vi "SymmetricalComponents_src.vi"(0 "A":T1, 5 "B":T1, 7 "C":T1) -> (4 "zero":T1, 6 "positive":T1, 8 "negative":T1)   [LabVIEW 2015]
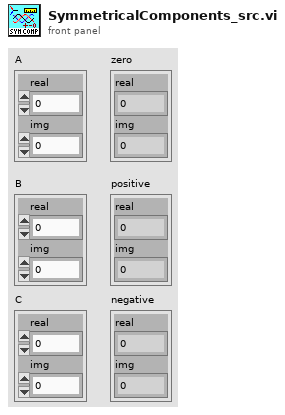
[diagram p1: front panel]
types:
  T1 = typedef "ComplexSGL" = cluster{"real":sgl, "img":sgl}
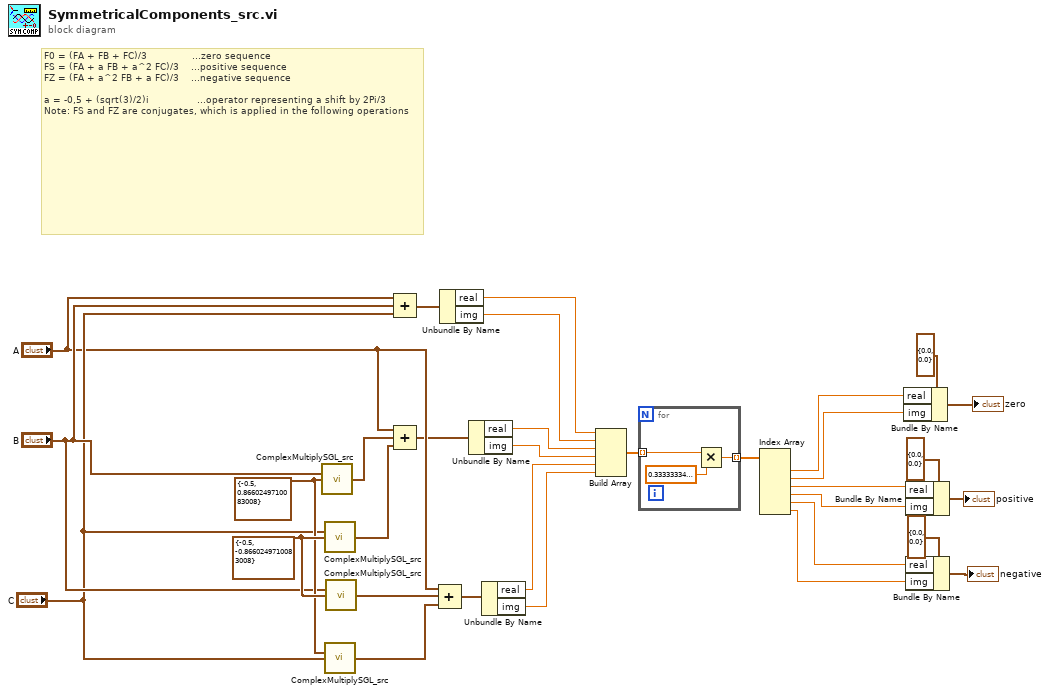
[diagram p0: block diagram]
diagram:
  w26 = T1 {"real"=-0.5, "img"=-0.866025} ("Y")
  w25 = T1 {"real"=-0.5, "img"=0.866025} ("Y")
  # "F0 = (FA + FB + FC)/3               ...zero sequence\nFS = (FA + a FB + a^2 FC)/3    ...positive sequence\nFZ = (FA + a^2 FB + a FC)/3    ...negative sequence\n\na = -0,5 + (sqrt(3)/2)i                ...operator representing a shift by 2Pi/3\nNote: FS and FZ are conjugates, which is applied in the following operations"
  n1 = call "ComplexMultiplySGL_src.vi"("X"="B", "Y"=w25) -> ("Z"=w11:T1)  [unwired: 13 in]
  n2 = call "ComplexMultiplySGL_src.vi"("X"="C", "Y"=w26) -> ("Z"=w10:T1)  [unwired: 13 in]
  n3 = call "ComplexMultiplySGL_src.vi"("X"=w25, "Y"="C") -> ("Z"=w7:T1)  [unwired: 13 in]
  n4 = call "ComplexMultiplySGL_src.vi"("X"="B", "Y"=w26) -> ("Z"=w8:T1)  [unwired: 13 in]
  n5 = Compound Arithmetic op=ADD("A", "B", "C") -> (w14:T1)
  n6 = Compound Arithmetic op=ADD("A", w11, w10) -> (w6:T1)
  n7 = Compound Arithmetic op=ADD("A", w8, w7) -> (w5:T1)
  n8 = Unbundle By Name(w14) -> ("real"=w13:sgl, "img"=w12:sgl)
  n9 = Unbundle By Name(w6) -> ("real"=w4:sgl, "img"=w3:sgl)
  n10 = Unbundle By Name(w5) -> ("real"=w2:sgl, "img"=w1:sgl)
  n11 = Build Array(w13, w12, w4, w3, w2, w1) -> (w32:sgl[])
  n12 = for {
    tunnel: w32 -> [w35] mode=indexing
    tunnel: [w33] -> w31 mode=indexing
    n13 = Multiply(x=w35, y=sgl 0.33333334) -> (x*y=w33:sgl)
  }
  n14 = Index Array(array=w31) -> (element #1=w30:sgl, element #2=w28:sgl, element #3=w20:sgl, element #4=w19:sgl, element #5=w18:sgl, element #6=w17:sgl)  [unwired: 6 in]
  n15 = Bundle By Name(cluster=T1 {"real"=0.0, "img"=0.0} ("zero"), "real"=w30, "img"=w28) -> (→"zero":T1)
  n16 = Bundle By Name(cluster=T1 {"real"=0.0, "img"=0.0} ("zero"), "real"=w20, "img"=w19) -> (→"positive":T1)
  n17 = Bundle By Name(cluster=T1 {"real"=0.0, "img"=0.0} ("zero"), "real"=w18, "img"=w17) -> (→"negative":T1)
